vi "Autosetup.vi"(8 "error in (no error)":errorcluster, 11 "VISA resource name":refnum<visa-resource-name>) -> (0 "error out":errorcluster, 3 "VISA resource name out":refnum<visa-resource-name>)   [LabVIEW 2015, in "Tektronix 7000 Series.lvlib"]
doc: "Configures the oscilloscope to evaluate all input waveforms and determine the optimum conditions for displaying the waveform. The Autosetup VI sets the oscilloscope to continuous acquisition mode."
uses:
  Tektronix 7000 Series.lvlib
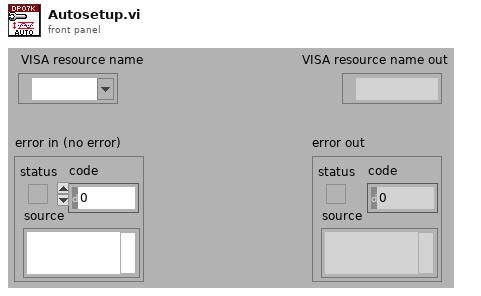
[diagram p1: front panel]
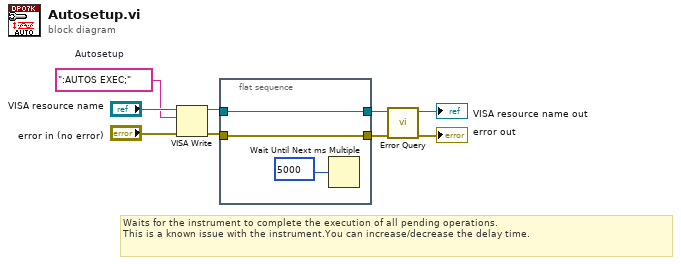
[diagram p0: block diagram]
diagram:
  w7 = ":AUTOS EXEC;"  # Autosetup
  # "Waits for the instrument to complete the execution of all pending operations.\nThis is a known issue with the instrument.You can increase/decrease the delay time."
  n1 = VISA Write(VISA resource name="VISA resource name", write buffer=w7, error in (no error)="error in (no error)") -> (VISA resource name out=w4:refnum<visa-resource-name>, error out=w3:errorcluster)  [unwired: 1 out]
  n2 = flat-sequence {
    tunnel: w4 -> [w12]
    tunnel: [w12] -> w2
    tunnel: w3 -> [w11]
    tunnel: [w11] -> w1
    frame #0 {
      n3 = Wait Until Next ms Multiple(millisecond multiple=u32 5000 ("Delay Time (5000ms)")) -> ()  [unwired: 1 out]
    }
  }
  n4 = call "Error Query.vi"("error in (no error)"=w1, "VISA resource name"=w2) -> ("error out"=→"error out":errorcluster, "VISA resource name out"=→"VISA resource name out":refnum<visa-resource-name>)  [unwired: 6 in, 2 out]
